vi "daemon.vi"(8 "error in (no error)":errorcluster, 11 "ComicVine_manager.lvclass":refnum<class "CV_downloader.lvclass">) -> ()   [LabVIEW 2024, in "CV_downloader.lvclass"]
uses:
  CV_downloader.lvclass
  CV_downloader.lvclass/CV_downloader.ctl
  states--enum.ctl
  <vilib>/addons/_JKI.lib/REST Client/classes/REST Client/REST Client.lvclass
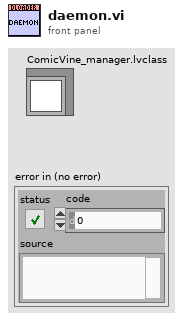
[diagram p1: front panel]
types:
  T1 = typedef "CV_downloader.lvclass/states--enum.ctl" = enum16{"start", "running", "start timer", "update file", "set directories", "wait", "shutdown"}
  T2 = cluster{"volume directory":path, "issue directory":path}
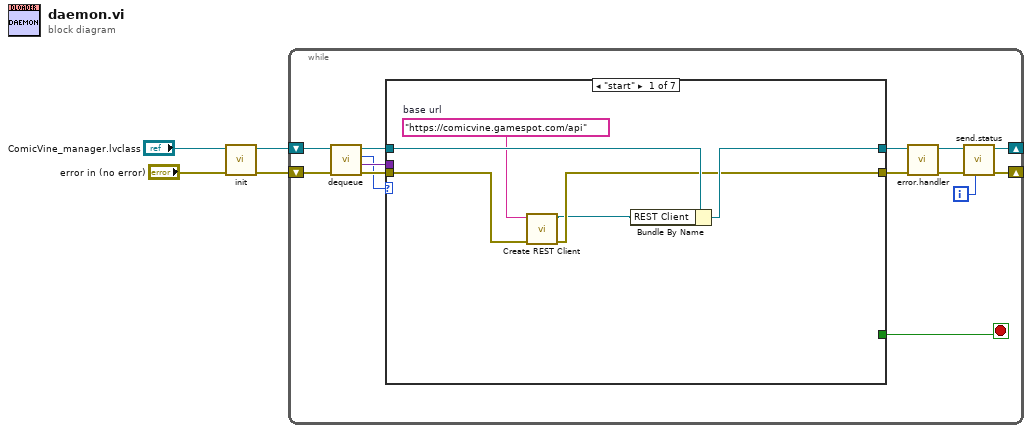
[diagram p0: block diagram]
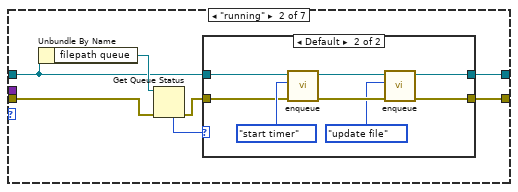
[diagram p2: hidden frame]
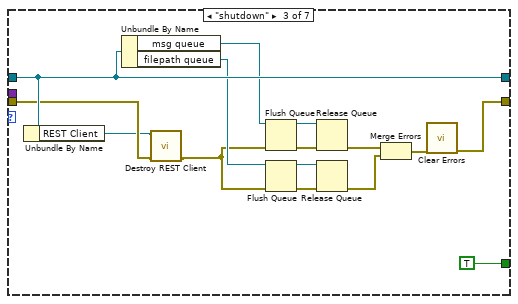
[diagram p4: hidden frame]
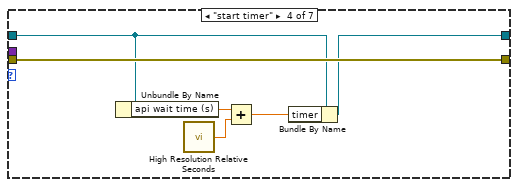
[diagram p5: hidden frame]
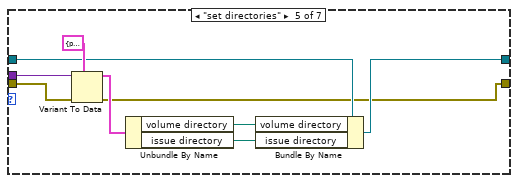
[diagram p6: hidden frame]
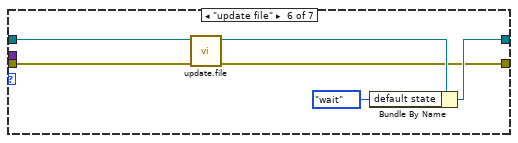
[diagram p7: hidden frame]
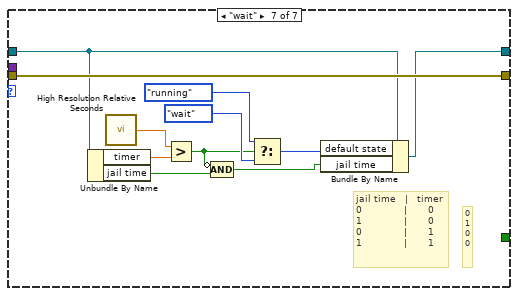
[diagram p8: hidden frame]
diagram:
  n1 = call "init.vi"("error in (no error)"="error in (no error)", "ComicVine_manager in"="ComicVine_manager.lvclass") -> ("error out"=w1:errorcluster, "ComicVine_manager out"=w3:refnum<class "CV_downloader.lvclass">)  [unwired: 8 in]
  n2 = while {
    shift-right: [w10] -> _
    shift-left: w3 -> [w18]
    shift-right: [w9] -> _
    shift-left: w1 -> [w17]
    i -> [w11]
    stop <- w12 stop-if-true
    n3 = call "dequeue.vi"("error in (no error)"=w17, "ComicVine_manager in"=w18) -> ("error out"=w16:errorcluster, "data"=w15:variant, "cmd"=w13:T1, "ComicVine_manager out"=w14:refnum<class "CV_downloader.lvclass">)  [unwired: 6 in]
    n4 = case shown="\"start\"" w13 {
      tunnel: w16 -> [w22 w30 w44 w62 w69 w72 w88]
      tunnel: w15 -> [_ _ _ _ w70 _ _]
      tunnel: w14 -> [w24 w28 w55 w59 w67 w74 w85]
      tunnel: [w23 w25 w55 w57 w64 w76 w81] -> w8
      tunnel: [w21 w26 w45 w62 w63 w73 w88] -> w7
      tunnel: [_ _ TRUE _ _ _ _] -> w12
      frame "start" {
        w19 = "https://comicvine.gamespot.com/api"  # base url
        n5 = call <vilib>:"Create REST Client.vi"("error in (no error)"=w22, "Base URL"=w19) -> ("error out"=w21:errorcluster, "REST Client out"=w20:refnum<class "REST Client.lvclass">)  [unwired: 8 in]
        n6 = Bundle By Name(cluster=w24, "REST Client"=w20) -> (w23:refnum<class "CV_downloader.lvclass">)
      }
      frame "running" {
        n7 = Unbundle By Name(w28) -> ("filepath queue"=w31:refnum<queue>)
        n8 = Get Queue Status(queue=w31, error in (no error)=w30) -> (error out=w27:errorcluster, # elements in queue=w29:i32)  [unwired: 1 in, 6 out]
        n9 = case shown="Default" w29 {
          tunnel: w28 -> [w32 w41]
          tunnel: w27 -> [w33 w39]
          tunnel: [w33 w37] -> w26
          tunnel: [w32 w35] -> w25
          frame 0 {
          }
          frame Default {
            n10 = call "enqueue.vi"("error in (no error)"=w39, "cmd"=states--enum."start timer" ("default state"), "ComicVine_manager in"=w41) -> ("error out"=w38:errorcluster, "ComicVine_manager out"=w36:refnum<class "CV_downloader.lvclass">)  [unwired: 7 in]
            n11 = call "enqueue.vi"("error in (no error)"=w38, "cmd"=states--enum."update file" ("default state"), "ComicVine_manager in"=w36) -> ("error out"=w37:errorcluster, "ComicVine_manager out"=w35:refnum<class "CV_downloader.lvclass">)  [unwired: 7 in]
          }
        }
      }
      frame "shutdown" {
        n12 = Unbundle By Name(w55) -> ("REST Client"=w42:refnum<class "REST Client.lvclass">)
        n13 = Unbundle By Name(w55) -> ("msg queue"=w52:refnum<queue>, "filepath queue"=w54:refnum<queue>)
        n14 = call-dynamic "Destroy REST Client.vi"("error in (no error)"=w44, "REST Client in"=w42) -> ("error out"=w43:errorcluster)  [unwired: 9 in]
        n15 = Flush Queue(queue=w52, error in (no error)=w43) -> (queue out=w51:refnum<queue>, error out=w50:errorcluster)  [unwired: 1 out]
        n16 = Flush Queue(queue=w54, error in (no error)=w43) -> (queue out=w53:refnum<queue>, error out=w47:errorcluster)  [unwired: 1 out]
        n17 = Release Queue(queue=w51, error in (no error)=w50) -> (error out=w49:errorcluster)  [unwired: 1 in, 2 out]
        n18 = Release Queue(queue=w53, error in (no error)=w47) -> (error out=w48:errorcluster)  [unwired: 1 in, 2 out]
        n19 = Merge Errors(w49, w48) -> (w46:errorcluster)
        n20 = call <vilib>:"Clear Errors.vi"("error in (no error)"=w46) -> ("error out"=w45:errorcluster)  [unwired: 5 in, 1 out]
      }
      frame "start timer" {
        n21 = Unbundle By Name(w59) -> ("api wait time (s)"=w61:dbl)
        n22 = call <vilib>:"High Resolution Relative Seconds.vi"() -> ("relative seconds"=w60:dbl)
        n23 = Add(x=w61, y=w60) -> (x+y=w58:dbl)
        n24 = Bundle By Name(cluster=w59, "timer"=w58) -> (w57:refnum<class "CV_downloader.lvclass">)
      }
      frame "set directories" {
        n25 = Variant To Data(error in=w69, type=T2 {"volume directory"=path "", "issue directory"=path ""}, Variant=w70) -> (data=w68:T2, error out=w63:errorcluster)
        n26 = Unbundle By Name(w68) -> ("volume directory"=w66:path, "issue directory"=w65:path)
        n27 = Bundle By Name(cluster=w67, "volume directory"=w66, "issue directory"=w65) -> (w64:refnum<class "CV_downloader.lvclass">)
      }
      frame "update file" {
        n28 = call "update.file.vi"("error in (no error)"=w72, "ComicVine_manager in"=w74) -> ("error out"=w73:errorcluster, "ComicVine_manager out"=w75:refnum<class "CV_downloader.lvclass">)  [unwired: 8 in]
        n29 = Bundle By Name(cluster=w75, "default state"=states--enum."wait") -> (w76:refnum<class "CV_downloader.lvclass">)
      }
      frame "wait" {
        # "0\n1\n0\n0"
        # "jail time   |   timer\n0              |       0\n1              |       0\n0              |       1\n1              |       1"
        n30 = Unbundle By Name(w85) -> ("timer"=w87:dbl, "jail time"=w78:bool)
        n31 = call <vilib>:"High Resolution Relative Seconds.vi"() -> ("relative seconds"=w86:dbl)
        n32 = Greater?(x=w86, y=w87) -> (0:w79:bool)
        n33 = Compound Arithmetic op=AND(invert w79, w78) -> (w80:bool)
        n34 = Select(t=states--enum."running" ("default state"), s=w79, f=states--enum."wait") -> (s? t:f=w82:T1)
        n35 = Bundle By Name(cluster=w85, "default state"=w82, "jail time"=w80) -> (w81:refnum<class "CV_downloader.lvclass">)
      }
    }
    n36 = call "error.handler.vi"("error in (no error)"=w7, "ComicVine_manager in"=w8) -> ("error out"=w6:errorcluster, "ComicVine_manager out"=w5:refnum<class "CV_downloader.lvclass">)  [unwired: 8 in]
    n37 = call "send.status.vi"("iteration"=w11, "error in (no error)"=w6, "ComicVine_manager in"=w5) -> ("error out"=w9:errorcluster, "ComicVine_manager out"=w10:refnum<class "CV_downloader.lvclass">)  [unwired: 7 in]
  }
